vi "test_ini - 1.vi"() -> ()   [LabVIEW 2016]
uses:
  <vilib>/Utility/config.llb/Write Key (Double).vi
  <vilib>/Utility/config.llb/Write Key (Boolean).vi
  <vilib>/Utility/config.llb/Read Key (Double).vi
  <vilib>/Utility/config.llb/Read Key (Boolean).vi
  <vilib>/Utility/config.llb/NI_LVConfig.lvlib
panel:
  in  "stop":bool
  in  "write":bool
  in  "read":bool
  in  "Slide":dbl(slide) scale=0.0..10.0
  in  "GAS":bool
  in  "I":dbl
  in  "U":dbl
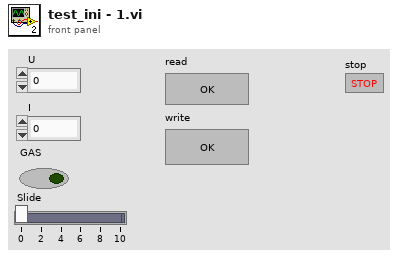
[diagram p1: front panel]
types:
  T1 = enum16{"open", "replace", "create", "open or create", "replace or create", "replace or create with confirmation"}
  T2 = typedef "NI_LVConfig.lvlib/Config Data RefNum.ctl" = refnum<k1>
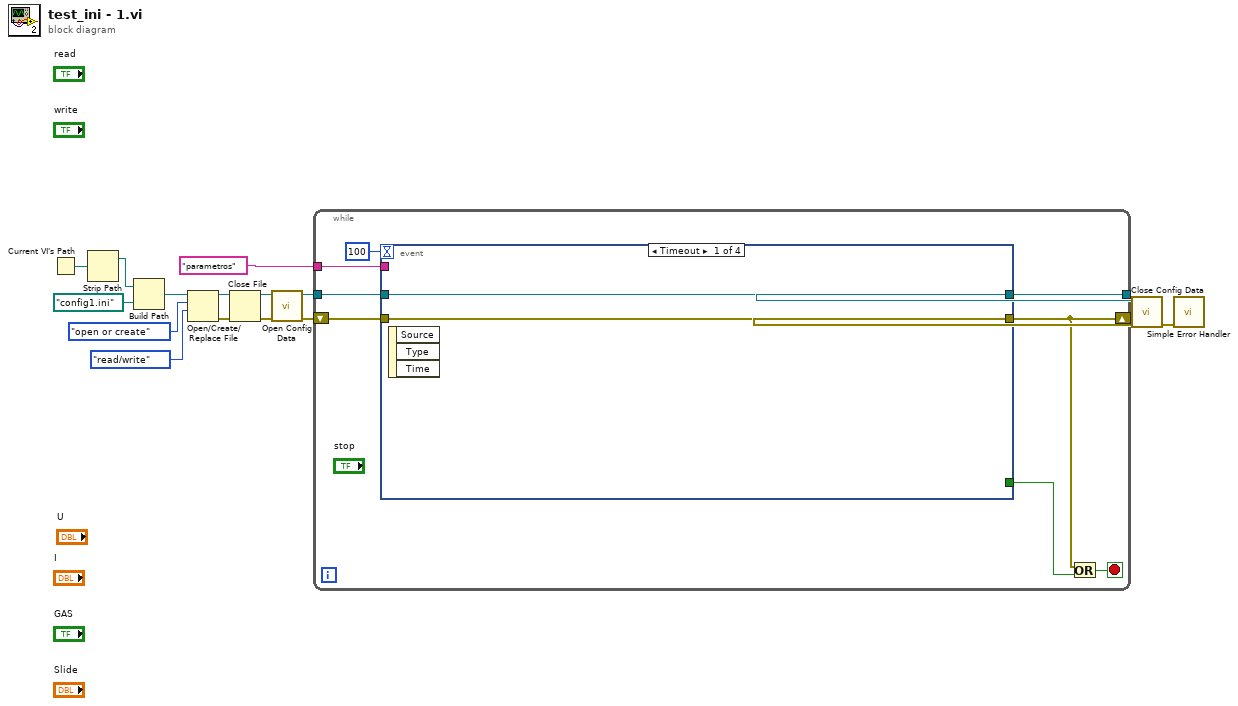
[diagram p0: block diagram]
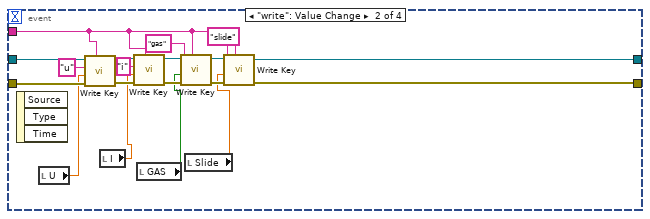
[diagram p2: hidden frame]
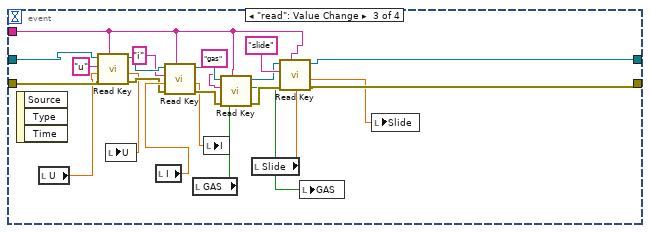
[diagram p3: hidden frame]
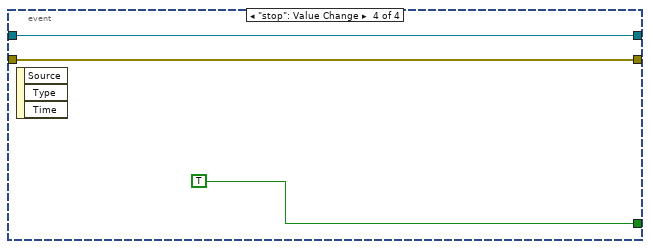
[diagram p4: hidden frame]
diagram:
  n1 = Current VI's Path() -> (path=w16:path)
  n2 = Strip Path(path=w16) -> (stripped path=w15:path)  [unwired: 1 out]
  n3 = Build Path(base path=w15, name or relative path=path "config1.ini") -> (appended path=w13:path)
  n4 = Open/Create/Replace File(file path (use dialog)=w13, operation (0:open)=T1."open or create", access (0:read/write)=enum16{"read/write", "read-only", "write-only"}."read/write") -> (refnum out=w10:refnum<file>, error out=w9:errorcluster)  [unwired: 3 in, 1 out]
  n5 = Close File(refnum=w10, error in=w9) -> (path=w8:path, error out=w1:errorcluster)
  n6 = call <vilib>:"Open Config Data.vi"("error in (no error)"=w1, "configuration file path"=w8) -> ("error out"=w6:errorcluster, "refnum"=w7:T2)  [unwired: 7 in, 1 out]
  n7 = while {
    shift-right: [w20] -> w5
    shift-left: w6 -> [w21]
    tunnel: w7 -> [w22]
    tunnel: [w19] -> w3
    tunnel: "parametros" ("section") -> [w17]
    stop <- w24 stop-if-true
    n8 = event shown="[0] Timeout" {
      selector: _ -> [_ _ _ _]
      dyn-events: _ -> [_ _ _ _]
      timeout: 100 -> [_ _ _ _]
      tunnel: w22 -> [w26 w45 w66 w71]
      tunnel: w21 -> [w25 w44 w67 w70]
      tunnel: [w25 w38 w63 w70] -> w20
      tunnel: [w26 w39 w64 w71] -> w19
      tunnel: [_ _ _ TRUE] -> w18
      tunnel: w17 -> [_ w27 w57 _]
      event Timeout {
        n9 = event-data() -> ()  [unwired: 1 in, 3 out]
      }
      event "write": Value Change {
        n10 = event-data() -> ()  [unwired: 1 in, 3 out]
        n11 = local read "U"() -> (w42:dbl)
        n12 = call-poly <vilib>:"Write Key.vi"("section"=w27, "error in (no error)"=w44, "value"=w42, "key"="u", "refnum"=w45) -> ("error out"=w40:errorcluster, "refnum out"=w41:T2)  [unwired: 4 in, 1 out]
        n13 = local read "I"() -> (w30:dbl)
        n14 = call-poly <vilib>:"Write Key.vi"("section"=w27, "error in (no error)"=w40, "value"=w30, "key"="i", "refnum"=w41) -> ("error out"=w34:errorcluster, "refnum out"=w35:T2)  [unwired: 4 in, 1 out]
        n15 = local read "GAS"() -> (w29:bool)
        n16 = call-poly <vilib>:"Write Key.vi"("section"=w27, "error in (no error)"=w34, "value"=w29, "key"="gas", "refnum"=w35) -> ("error out"=w37:errorcluster, "refnum out"=w36:T2)  [unwired: 4 in, 1 out]
        n17 = local read "Slide"() -> (w28:dbl)
        n18 = call-poly <vilib>:"Write Key.vi"("section"=w27, "error in (no error)"=w37, "value"=w28, "key"="slide", "refnum"=w36) -> ("error out"=w38:errorcluster, "refnum out"=w39:T2)  [unwired: 4 in, 1 out]
      }
      event "read": Value Change {
        n19 = event-data() -> ()  [unwired: 1 in, 3 out]
        n20 = local read "U"() -> (w65:dbl)
        n21 = call-poly <vilib>:"Read Key.vi"("section"=w57, "error in (no error)"=w67, "default value"=w65, "key"="u", "refnum"=w66) -> ("error out"=w59:errorcluster, "value"=w49:dbl, "refnum out"=w60:T2)  [unwired: 3 in, 1 out]
        n22 = local write "U"(w49) -> ()
        n23 = local read "I"() -> (w61:dbl)
        n24 = call-poly <vilib>:"Read Key.vi"("section"=w57, "error in (no error)"=w59, "default value"=w61, "key"="i", "refnum"=w60) -> ("error out"=w53:errorcluster, "value"=w48:dbl, "refnum out"=w54:T2)  [unwired: 3 in, 1 out]
        n25 = local read "GAS"() -> (w51:bool)
        n26 = local write "I"(w48) -> ()
        n27 = call-poly <vilib>:"Read Key.vi"("section"=w57, "error in (no error)"=w53, "default value"=w51, "key"="gas", "refnum"=w54) -> ("error out"=w56:errorcluster, "found?"=w47:bool, "refnum out"=w55:T2)  [unwired: 3 in, 1 out]
        n28 = local read "Slide"() -> (w50:dbl)
        n29 = call-poly <vilib>:"Read Key.vi"("section"=w57, "error in (no error)"=w56, "default value"=w50, "key"="slide", "refnum"=w55) -> ("error out"=w63:errorcluster, "value"=w46:dbl, "refnum out"=w64:T2)  [unwired: 3 in, 1 out]
        n30 = local write "GAS"(w47) -> ()
        n31 = local write "Slide"(w46) -> ()
      }
      event "stop": Value Change {
        n32 = event-data() -> ()  [unwired: 1 in, 3 out]
      }
    }
    n33 = Or(x=w20, y=w18) -> (x .or. y?=w24:bool)
  }
  n34 = call <vilib>:"Close Config Data.vi"("error in (no error)"=w5, "refnum"=w3) -> ("error out"=w4:errorcluster)  [unwired: 8 in, 1 out]
  n35 = call <vilib>:"Simple Error Handler.vi"("error in (no error)"=w4) -> ()  [unwired: 4 in, 5 out]
